vi "My_Subscript.vi"() -> ()   [LabVIEW 2019]
uses:
  <vilib>/LabVIEW Open Source Project/MQTT Client/Client class/Client.lvclass/Client.ctl
  <vilib>/LabVIEW Open Source Project/MQTT Connection/MQTT_Base/Base Class/MQTT_Base.lvclass/MQTT_Base.ctl
  <vilib>/LabVIEW Open Source Project/MQTT TCP Connection/MQTT_TCP/Connection/TCPConnection.lvclass
  C:/Program Files (x86)/National Instruments/LabVIEW 2019/vi.lib/LabVIEW Open Source Project/MQTT Connection/MQTT_Connection/Connection/Connection.lvclass
  <vilib>/LabVIEW Open Source Project/MQTT Client/Client class/Client.lvclass
  C:/Program Files (x86)/National Instruments/LabVIEW 2019/vi.lib/LabVIEW Open Source Project/MQTT Connection/MQTT_Base/Base Class/MQTT_Base.lvclass
  <vilib>/LabVIEW Open Source Project/MQTT Control Packets/Control Packets/PUBLISH/PUBLISH.lvclass
  <vilib>/LabVIEW Open Source Project/MQTT Connection/MQTT_Base/Base Class/MQTT_Base.lvclass
panel:
  out "Unsuback":bool
  out "Suback":bool
  in  "Subscribe":bool
  in  "Connection":bool
  in  "Stop Client":bool
  out "Waveform Chart":dbl(graph)
  out "last error":errorcluster
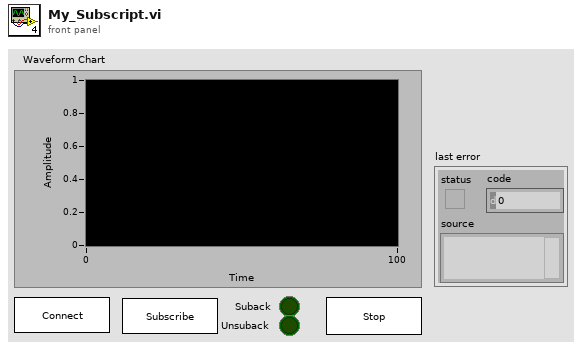
[diagram p1: front panel]
types:
  T1 = typedef "MQTT Client.lvlib/Client.lvclass/Public Events -- cluster.ctl" = cluster{"Connection Status":refnum<user-event>, "Connected":refnum<user-event>, "Application Message":refnum<user-event>}
  T2 = typedef "MQTT Base.lvlib/MQTT_Base.lvclass/Public Events -- cluster.ctl" = cluster{"Stop Event":refnum<user-event>, "Error Event":refnum<user-event>, "Inbound Message":refnum<user-event>}
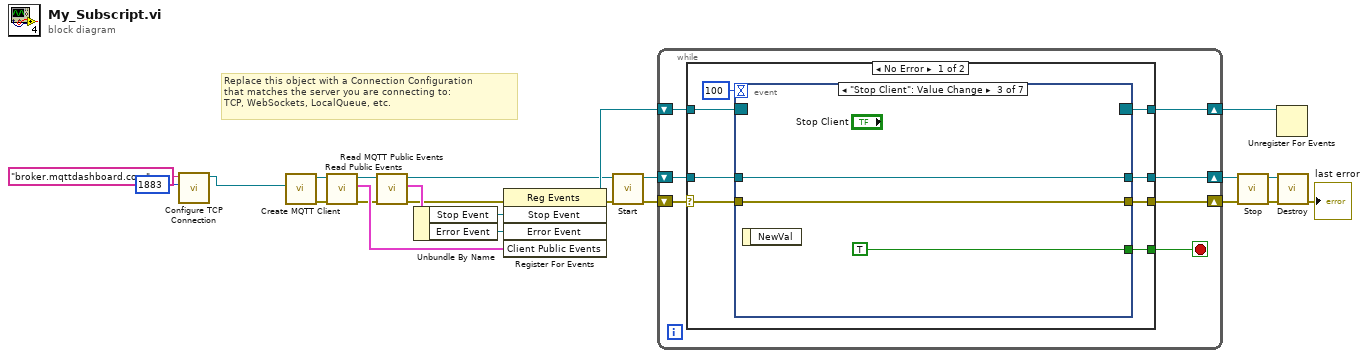
[diagram p0: block diagram]
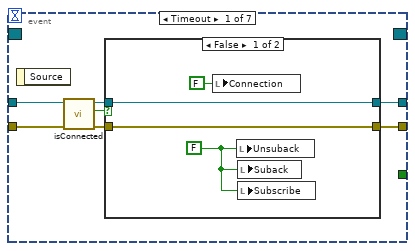
[diagram p2: hidden frame]
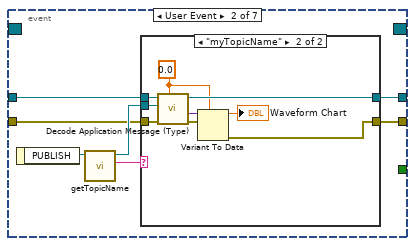
[diagram p4: hidden frame]
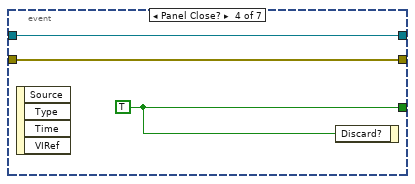
[diagram p6: hidden frame]
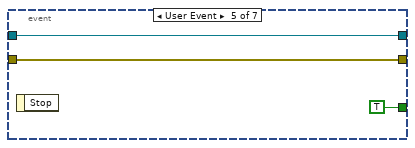
[diagram p7: hidden frame]
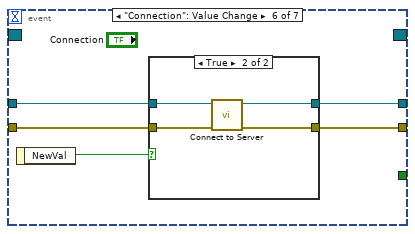
[diagram p8: hidden frame]
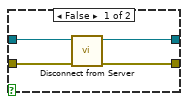
[diagram p9: hidden frame]
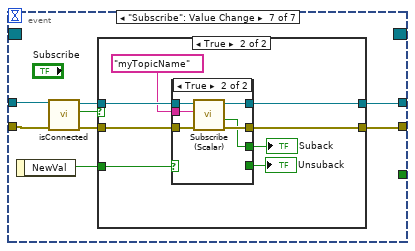
[diagram p10: hidden frame]
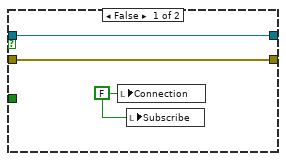
[diagram p11: hidden frame]
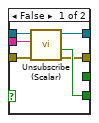
[diagram p12: hidden frame]
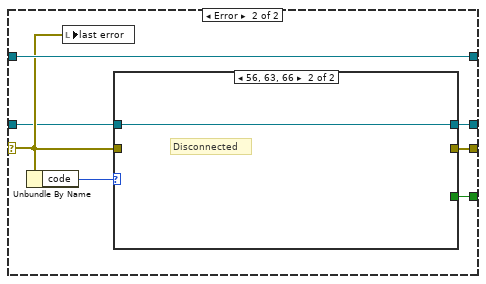
[diagram p13: hidden frame]
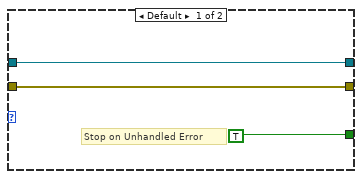
[diagram p14: hidden frame]
diagram:
  # "Replace this object with a Connection Configuration\nthat matches the server you are connecting to:\nTCP, WebSockets, LocalQueue, etc."
  n1 = call <vilib>:"Configure TCP Connection.vi"("remote port (80)"=u16 1883, "address (localhost)"="broker.mqttdashboard.com") -> ("TCPConnection"=w3:refnum<class "TCPConnection.lvclass">)  [unwired: 8 in, 1 out]
  n2 = call <vilib>:"Create MQTT Client.vi"("Connection Configuration"=w3) -> ("error out"=w6:errorcluster, "Client out"=w4:refnum<class "Client.lvclass">)  [unwired: 9 in]
  n3 = call <vilib>:"Read Public Events.vi"("error in (no error)"=w6, "Client in"=w4) -> ("error out"=w7:errorcluster, "Client Public Events"=w9:T1, "Client out"=w5:refnum<class "Client.lvclass">)  [unwired: 7 in]
  n4 = call <vilib>:"Read MQTT Public Events.vi"("error in (no error)"=w7, "MQTT_Base in"=w5) -> ("error out"=w8:errorcluster, "MQTT Public Events"=w16:T2, "MQTT_Base out"=w11:refnum<class "Client.lvclass">)  [unwired: 7 in]
  n5 = Unbundle By Name(w16) -> ("Stop Event"=w14:refnum<user-event>, "Error Event"=w15:refnum<user-event>)
  n6 = register-events(error in=w8, w14, w15, w9) -> (reference out=w12:refnum<event-registration>, error out=w10:errorcluster)  [unwired: 1 in]
  n7 = call <vilib>:"Start.vi"("error in (no error)"=w10, "MQTT_Base in"=w11) -> ("error out"=w22:errorcluster, "MQTT_Base out"=w21:refnum<class "Client.lvclass">)  [unwired: 7 in, 1 out]
  n8 = while {
    shift-right: [w29] -> w13
    shift-left: w12 -> [w30]
    shift-right: [w26] -> w18
    shift-left: w21 -> [w27]
    shift-right: [w28] -> w20
    shift-left: w22 -> [w24]
    stop <- w25 stop-if-true
    n9 = case shown="No Error" w24 {
      selector: w24 -> [w31 w126]
      tunnel: w30 -> [w38 w129]
      tunnel: [w37 w129] -> w29
      tunnel: [w36 w124] -> w28
      tunnel: w27 -> [w34 w125]
      tunnel: [w33 w128] -> w26
      tunnel: [w32 w123] -> w25
      frame No Error {
        n10 = event shown="[2] \"Stop Client\": Value Change" {
          selector: w38 -> [_ _ _ _ _ _ _]
          dyn-events: [_ _ _ _ _ _ _] -> w37
          timeout: 100 -> [_ _ _ _ _ _ _]
          tunnel: w31 -> [w41 w55 w71 w73 w78 w79 w97]
          tunnel: [w44 w52 w71 w73 w78 w80 w98] -> w36
          tunnel: [_ _ TRUE w75 TRUE _ _] -> w32
          tunnel: w34 -> [w43 w56 w72 w74 w76 w83 w96]
          tunnel: [w45 w54 w72 w74 w76 w81 w99] -> w33
          event Timeout {
            n11 = event-data() -> ()  [unwired: 1 in, 1 out]
            n12 = call <vilib>:"isConnected.vi"("error in (no error)"=w41, "Client in"=w43) -> ("error out"=w40:errorcluster, "connected"=w39:bool, "Client out"=w42:refnum<class "Client.lvclass">)  [unwired: 7 in]
            n13 = case shown="False" w39 {
              tunnel: [w49 w51] -> w45
              tunnel: [w48 w50] -> w44
              tunnel: w42 -> [w49 w51]
              tunnel: w40 -> [w48 w50]
              frame False {
                w47 = FALSE
                n14 = local write "Connection"(FALSE ("Connection")) -> ()
                n15 = local write "Unsuback"(w47) -> ()
                n16 = local write "Suback"(w47) -> ()
                n17 = local write "Subscribe"(w47) -> ()
              }
              frame True {
              }
            }
          }
          event User Event {
            n18 = event-data() -> ("PUBLISH"=w58:refnum<class "PUBLISH.lvclass">)  [unwired: 1 in]
            n19 = call <vilib>:"getTopicName.vi"("PUBLISH in"=w58) -> ("Topic"=w53:string, "PUBLISH out"=w57:refnum<class "PUBLISH.lvclass">)  [unwired: 8 in, 1 out]
            n20 = case shown="\"myTopicName\"" w53 {
              tunnel: w57 -> [_ w61]
              tunnel: w56 -> [w60 w67]
              tunnel: w55 -> [w59 w65]
              tunnel: [w60 w66] -> w54
              tunnel: [w59 w69] -> w52
              frame Default {
              }
              frame "myTopicName" {
                w63 = 0.0
                n21 = call <vilib>:"Decode Application Message (Type).vi"("Type"=w63, "error in (no error)"=w65, "PUBLISH"=w61, "Client in"=w67) -> ("error out"=w64:errorcluster, "Payload"=w62:variant, "Client out"=w66:refnum<class "Client.lvclass">)  [unwired: 4 in, 1 out]
                n22 = Variant To Data(error in=w64, type=w63, Variant=w62) -> (data=→"Waveform Chart":dbl, error out=w69:errorcluster)
              }
            }
          }
          event "Stop Client": Value Change {
            n23 = event-data() -> ()  [unwired: 1 in, 1 out]
          }
          event Panel Close? {
            w75 = TRUE
            n24 = event-data() -> ()  [unwired: 1 in, 4 out]
            n25 = event-data("Discard?"=w75) -> ()  [unwired: 1 in, 1 out]
          }
          event User Event {
            n26 = event-data() -> ()  [unwired: 1 in, 1 out]
          }
          event "Connection": Value Change {
            n27 = event-data() -> ("NewVal"=w82:bool)  [unwired: 1 in]
            n28 = case shown="True" w82 {
              tunnel: w83 -> [w87 w91]
              tunnel: [w86 w88] -> w81
              tunnel: [w85 w89] -> w80
              tunnel: w79 -> [w84 w90]
              frame False {
                n29 = call <vilib>:"Disconnect from Server.vi"("error in (no error)"=w84, "Client in"=w87) -> ("error out"=w85:errorcluster, "Client out"=w86:refnum<class "Client.lvclass">)  [unwired: 7 in, 1 out]
              }
              frame True {
                n30 = call <vilib>:"Connect to Server.vi"("error in (no error)"=w90, "Client in"=w91) -> ("error out"=w89:errorcluster, "Client out"=w88:refnum<class "Client.lvclass">)  [unwired: 6 in, 2 out]
              }
            }
          }
          event "Subscribe": Value Change {
            n31 = event-data() -> ("NewVal"=w92:bool)  [unwired: 1 in]
            n32 = call <vilib>:"isConnected.vi"("error in (no error)"=w97, "Client in"=w96) -> ("error out"=w94:errorcluster, "connected"=w93:bool, "Client out"=w95:refnum<class "Client.lvclass">)  [unwired: 7 in]
            n33 = case shown="True" w93 {
              tunnel: [w102 w110] -> w99
              tunnel: [w101 w109] -> w98
              tunnel: w95 -> [w102 w108]
              tunnel: w94 -> [w101 w107]
              tunnel: w92 -> [_ w105]
              frame False {
                w100 = FALSE ("Connection")
                n34 = local write "Connection"(w100) -> ()
                n35 = local write "Subscribe"(w100) -> ()
              }
              frame True {
                n36 = case shown="True" w105 {
                  tunnel: [w111 w119] -> w110
                  tunnel: [w112 w118] -> w109
                  tunnel: w108 -> [w116 w122]
                  tunnel: w107 -> [w115 w121]
                  tunnel: "myTopicName" ("Topic Name (empty: Payload name)") -> [w114 w120]
                  tunnel: [_ w117] -> w104
                  tunnel: [w113 _] -> w103
                  frame False {
                    n37 = call <vilib>:"Unsubscribe (Scalar).vi"("error in (no error)"=w115, "Topic Filter"=w114, "Client in"=w116) -> ("error out"=w112:errorcluster, "Ack"=w113:bool, "Client out"=w111:refnum<class "Client.lvclass">)  [unwired: 6 in]
                  }
                  frame True {
                    n38 = call <vilib>:"Subscribe (Scalar).vi"("error in (no error)"=w121, "Topic Filter"=w120, "Client in"=w122) -> ("error out"=w118:errorcluster, "Ack"=w117:bool, "Client out"=w119:refnum<class "Client.lvclass">)  [unwired: 6 in]
                  }
                }
                "Unsuback" <- w103
                "Suback" <- w104
              }
            }
          }
        }
      }
      frame Error {
        n39 = Unbundle By Name(w126) -> ("code"=w127:i32)
        n40 = local write "last error"(w126) -> ()
        n41 = case shown="56, 63, 66" w127 {
          tunnel: w125 -> [w132 w133]
          tunnel: [w132 w133] -> w128
          tunnel: w126 -> [w131 _]
          tunnel: [w131 _] -> w124
          tunnel: [TRUE _] -> w123
          frame Default {
            # "Stop on Unhandled Error"
          }
          frame 56, 63, 66 {
            # "Disconnected"
          }
        }
      }
    }
  }
  n42 = call <vilib>:"Stop.vi"("error in (no error)"=w20, "MQTT_Base in"=w18) -> ("error out"=w19:errorcluster, "MQTT_Base out"=w17:refnum<class "Client.lvclass">)  [unwired: 7 in, 1 out]
  n43 = Unregister For Events(event registration refnum=w13) -> ()  [unwired: 1 in, 1 out]
  n44 = call <vilib>:"Destroy.vi"("error in (no error)"=w19, "MQTT_Base in"=w17) -> ("error out"=→"last error":errorcluster)  [unwired: 8 in, 1 out]
